vi "2D Array to BMP.vi"(4 "2D color array":u32[][](array[numeric])) -> (1 "image data":T1)   [LabVIEW 2013]
uses:
  <vilib>/picture/picture.llb/imagedata.ctl
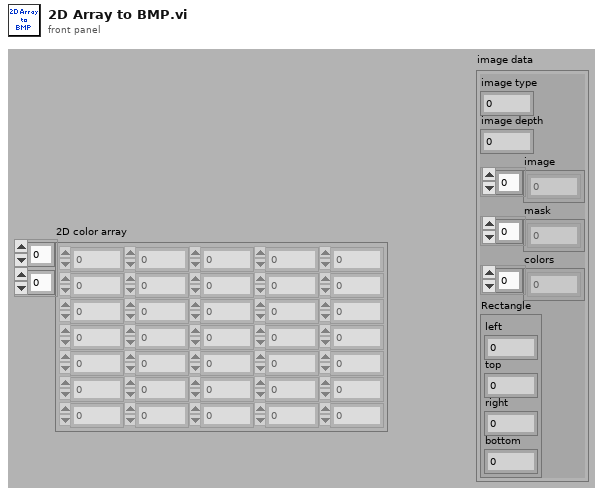
[diagram p1: front panel]
types:
  T1 = typedef "imagedata.ctl" = cluster{"image type":i32, "image depth":i32, "image":u8[], "mask":u8[], "colors":u32[], "Rectangle":cluster{"left":i16, "top":i16, "right":i16, "bottom":i16}}
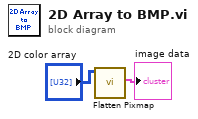
[diagram p0: block diagram]
diagram:
  n1 = call <vilib>:"Flatten Pixmap.vi"("24-bit pixmap"="2D color array") -> ("image data"=→"image data":T1)  [unwired: 10 in]
